vi "Ver 4.0.vi"() -> ()   [LabVIEW 2016]
doc: "This example VI shows how to use thermocouples to take a temperature measurement.\n\nNote:\nFor front panel measurements, make sure the Input switch is in the out position(F)\nFor plug-in card measurements, make sure the Input switch is in the in poisition(R)"
uses:
  Documents/keithley_27xx/Keithley 27XX/Public/Configure/Measurement Specific/Configure FRTD.vi
  Documents/keithley_27xx/Keithley 27XX/Public/Configure/Measurement Specific/Configure Thermocouple.vi
  Documents/keithley_27xx/Keithley 27XX/Public/Configure/Measurement Specific/Configure Thermistor.vi
  Documents/keithley_27xx/Keithley 27XX/Public/Data/Read Multiple Direct.vi
  Documents/keithley_27xx/Keithley 27XX/Keithley 27XX.lvlib
panel:
  out "XY Graph":cluster{dbl[], dbl[]}[](graph)
  out "Timestamp 2":dbl[](array[numeric])
  out "Timestamp 1":dbl[](array[numeric])
  out "Timestamp 0":dbl[](array[numeric])
  out "Case 2":dbl[](array[numeric])
  out "Case 1":dbl[](array[numeric])
  in  "Channel (2)":string="103"
  in  "Alpha2":dbl=0.0038
  in  "Beta2":dbl=0.1
  in  "Delta2 3":dbl=1.0
  in  "Sensor Type 2":string(combo)="Thermistor"
  in  "Channel (1)":string="102"
  in  "Alpha1":dbl=0.0038
  in  "Beta1":dbl=0.1
  in  "Delta1 2":dbl=1.0
  in  "Sensor Type 1":string(combo)="Thermistor"
  in  "Sensor Type 0":string(combo)="Thermistor"
  in  "Delta0":dbl=1.0
  in  "Beta0":dbl=0.1
  in  "Alpha0":dbl=0.0038
  in  "Serial Configuration":T1={"Baud Rate (9600)"=9600, "Flow Control (1: XON/XOFF)"=1, "Termination Char (0:CR)"=0} {"Termination Char (0:CR)" items=["CR", "LF", "CRLF (Do not use)", "LFCR (Do not use)"]; "Flow Control (1: XON/XOFF)" items=["None", "XON/XOFF", "RTS/CTS (2701 Only)", "XON/XOFF & RTS/CTS (2701 Only)"]; "Baud Rate (9600)" items=["300"=300, "600"=600, "1200"=1200, "2400"=2400, "4800"=4800, "9600"=9600, "19.2k"=19200, "38.4k (2701 Only)"=38400, "57.6k (2701 Only)"=57600, "115.2k (2701 Only)"=115200]}
  in  "VISA resource name":refnum<visa-resource-name>="TCPIP0::192.168.69.200::1394::SOCKET"
  in  "stop":bool
  out "Case 0":dbl[](array[numeric])
  in  "Channel (0)":string="101"
  in  "Temperature (0: Celsius)":u16(ring) items=["Celsius", "Fahrenheit", "Kelvin"]
  # "*For front panel measurements, make sure the Input switch is in the out position(F)*\n  For plug-in card measurements, make sure the Input switch is in the in position(R)"
  # "© 2005 National Instruments Corporation.  ALL RIGHTS RESERVED."
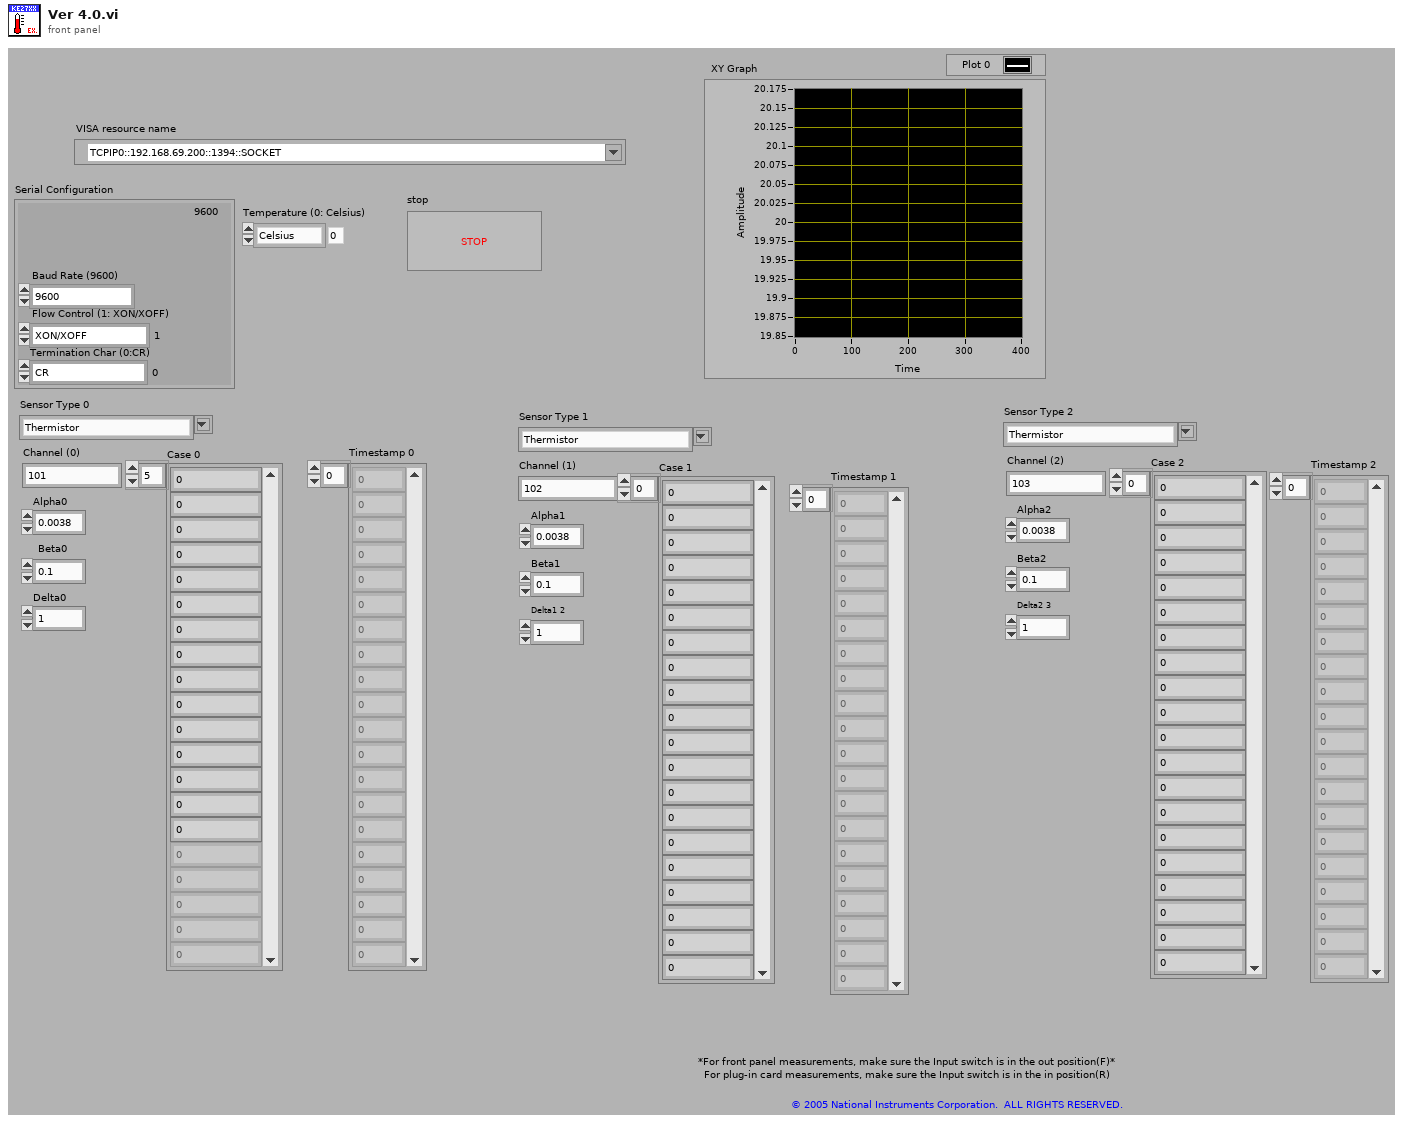
[diagram p1: front panel]
types:
  T1 = cluster{"Baud Rate (9600)":u32, "Flow Control (1: XON/XOFF)":u16, "Termination Char (0:CR)":u16}
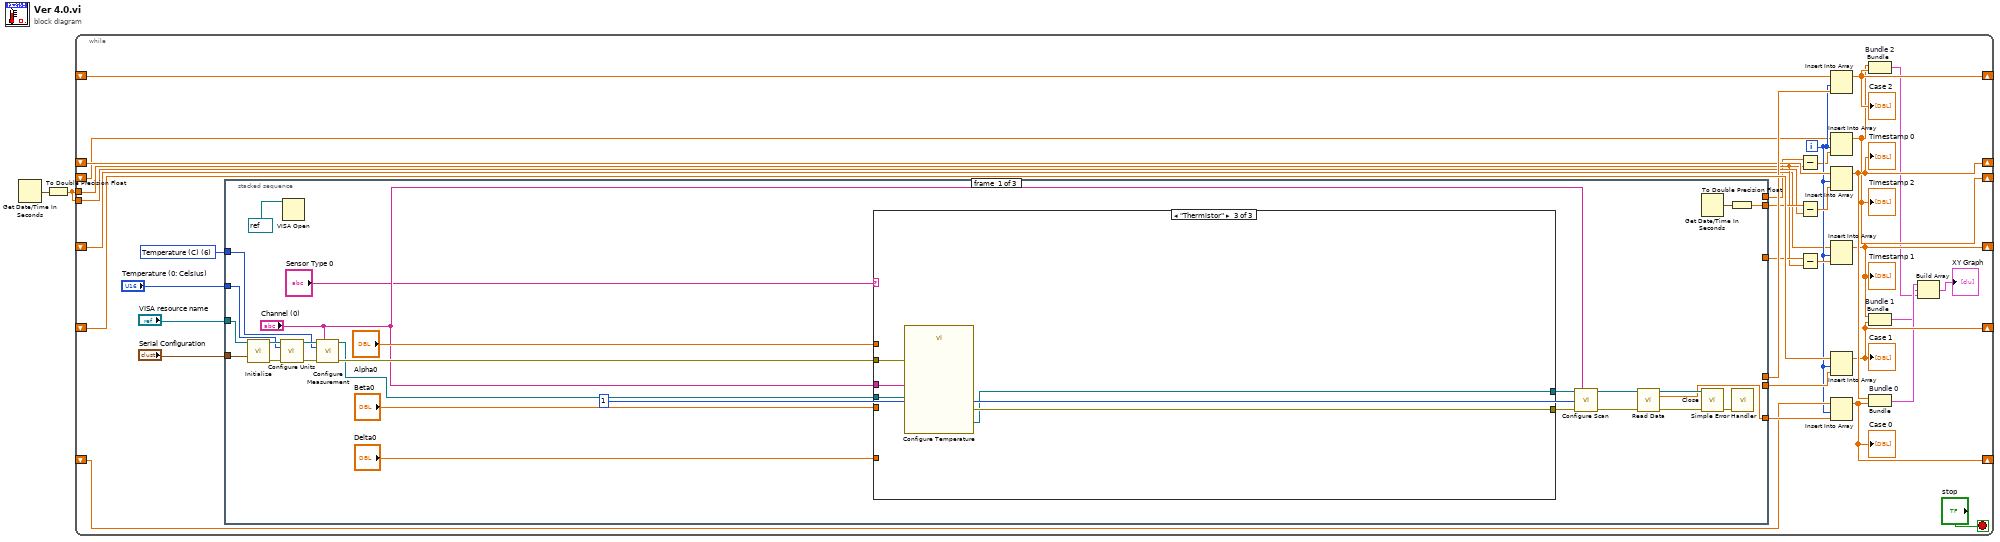
[diagram p0: block diagram]
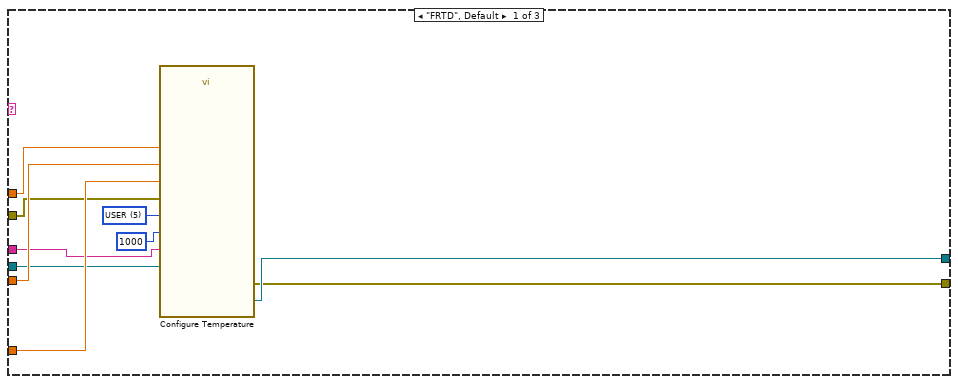
[diagram p2: hidden frame]
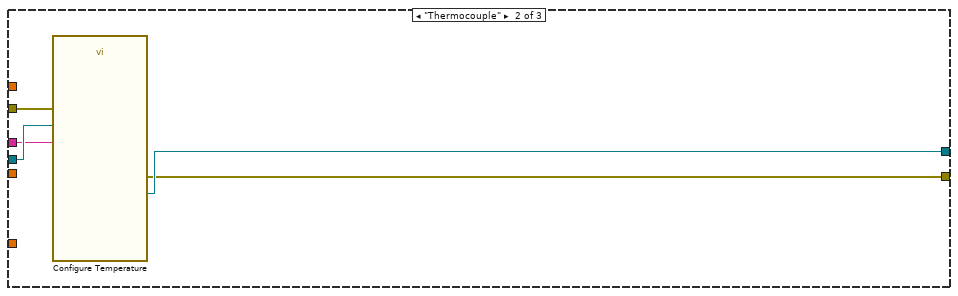
[diagram p3: hidden frame]
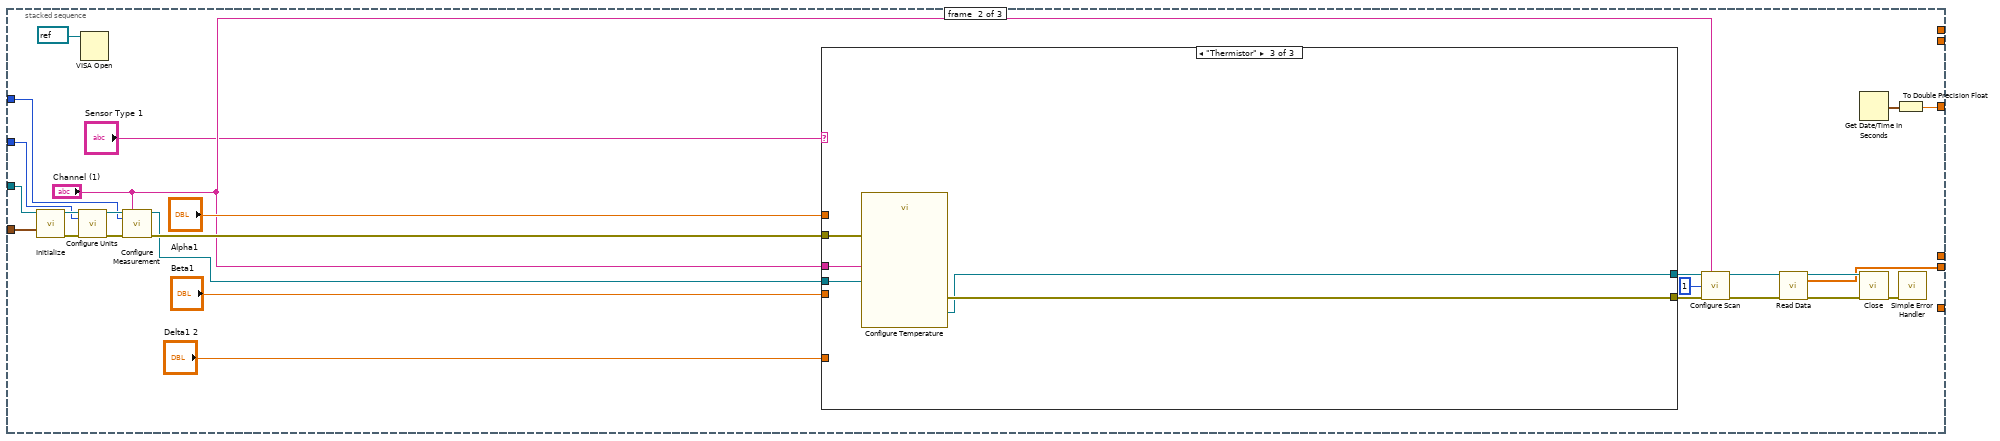
[diagram p4: hidden frame]
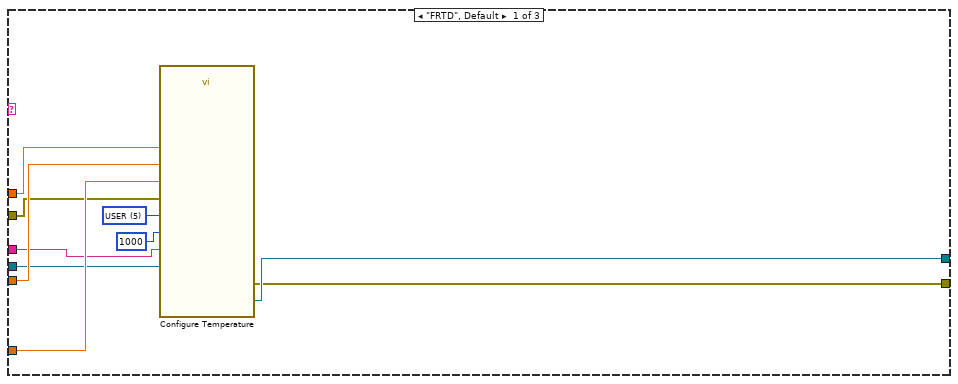
[diagram p5: hidden frame]
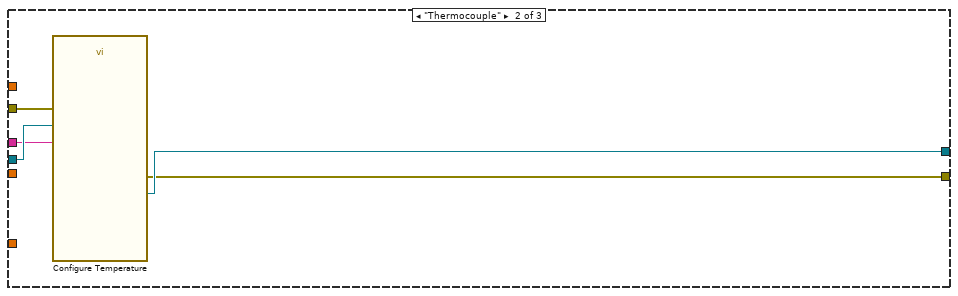
[diagram p6: hidden frame]
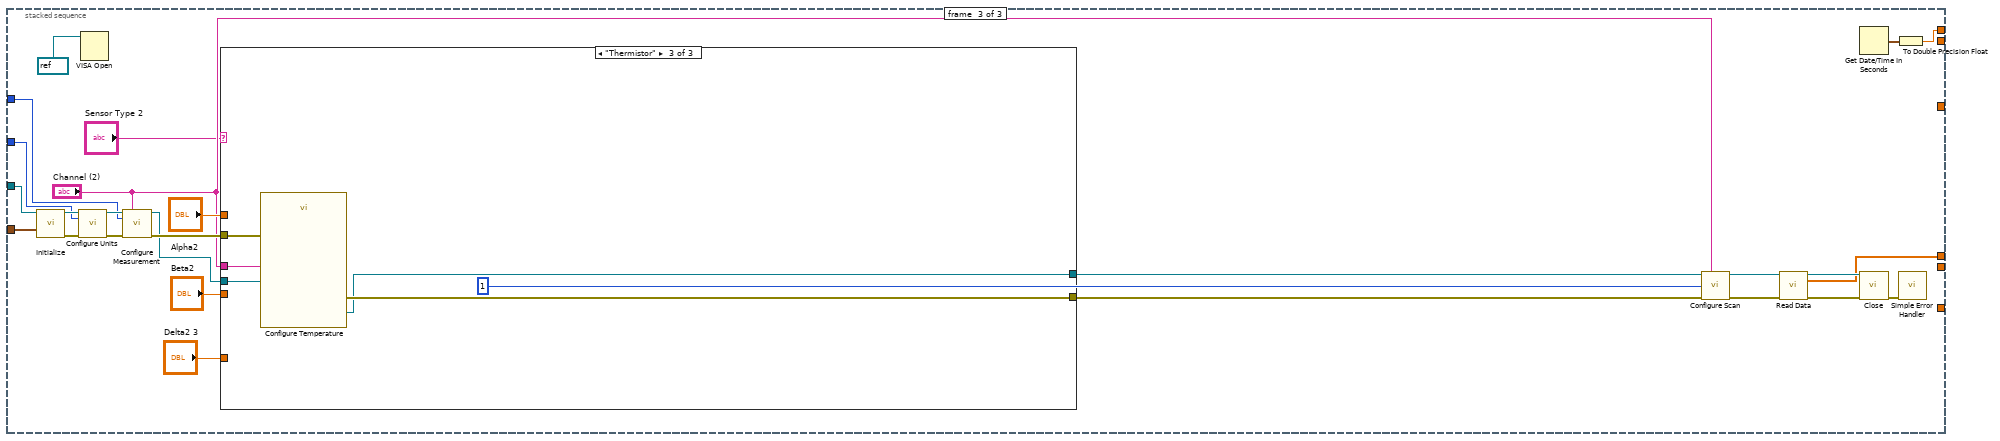
[diagram p7: hidden frame]
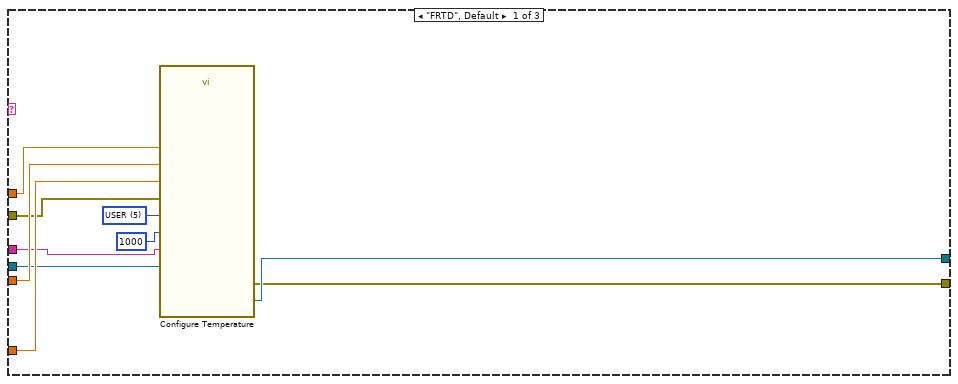
[diagram p8: hidden frame]
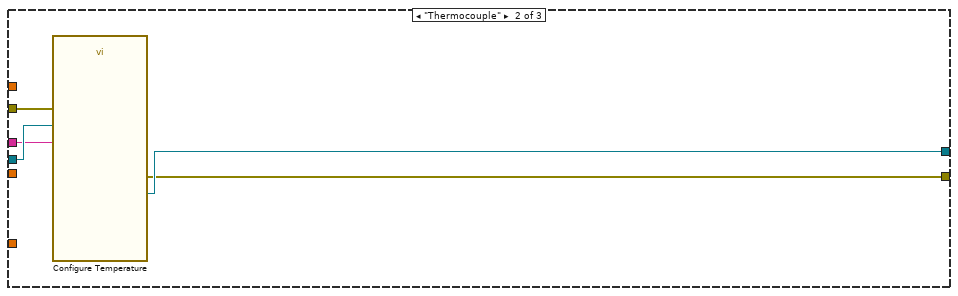
[diagram p9: hidden frame]
diagram:
  n1 = Get Date/Time In Seconds() -> (seconds since 1Jan1904=w2:timestamp)
  n2 = To Double Precision Float(number=w2) -> (double precision float=w1:dbl)
  n3 = while {
    shift-right: [w20] -> _
    shift-left: _ -> [w29]
    shift-right: [w11] -> _
    shift-left: _ -> [w27]
    shift-right: [w10] -> _
    shift-left: _ -> [w25]
    tunnel: w1 -> [w23]
    shift-right: [w19] -> _
    shift-left: _ -> [w21]
    tunnel: w1 -> [w17]
    shift-right: [w12] -> _
    shift-left: _ -> [w13]
    shift-right: [w9] -> _
    shift-left: _ -> [w8]
    i -> [w15]
    stop <- "stop" stop-if-true
    w33 = u16 6 items=["DC Voltage", "AC Voltage", "DC Current", "AC Current", "Resistance", "Four-Wire Resistance", "Temperature (C)", "Frequency", "Period", "Continuity"] ("Function (0: DC Voltage)")
    n4 = stacked-sequence {
      tunnel: "VISA resource name" -> [w52 w99 w146]
      tunnel: "Serial Configuration" -> [w51 w98 w145]
      tunnel: w33 -> [w50 w97 w144]
      tunnel: "Temperature (0: Celsius)" -> [w49 w96 w143]
      tunnel: [w38 _ _] -> w31
      tunnel: [_ w85 _] -> w28
      tunnel: [_ _ w132] -> w26
      tunnel: [w36 _ _] -> w24
      tunnel: [_ w83 _] -> w18
      tunnel: [_ _ w130] -> w7
      frame #0 {
        n5 = call "Initialize.vi"("VISA resource name"=w52, "Serial Configuration"=w51) -> ("VISA resource name out"=w61:refnum<visa-resource-name>, "error out"=w55:errorcluster)  [unwired: 12 in]
        n6 = call "Configure Units.vi"("VISA resource name"=w61, "Temperature (0: Celsius)"=w49, "error in (no error)"=w55) -> ("VISA resource name out"=w62:refnum<visa-resource-name>, "error out"=w54:errorcluster)  [unwired: 11 in]
        n7 = VISA Open(VISA resource name=refnum<visa-resource-name> refnum) -> ()  [unwired: 4 in, 2 out]
        n8 = call "Configure Measurement.vi"("VISA resource name"=w62, "Scan List (Empty)"="Channel (0)", "Function (0: DC Voltage)"=w50, "error in (no error)"=w54) -> ("VISA resource name out"=w42:refnum<visa-resource-name>, "error out"=w43:errorcluster)  [unwired: 10 in]
        n9 = case shown="\"Thermistor\"" "Sensor Type 0" {
          tunnel: [w71 w76 w82] -> w48
          tunnel: [w72 w77 w81] -> w47
          tunnel: "Delta0" -> [w66 _ _]
          tunnel: "Beta0" -> [w67 _ _]
          tunnel: "Alpha0" -> [w68 _ _]
          tunnel: w43 -> [w65 w75 w78]
          tunnel: w42 -> [w64 w74 w79]
          tunnel: "Channel (0)" -> [w63 w73 w80]
          frame "FRTD", Default {
            w70 = u16 5 items=["PT100", "D100", "F100", "PT3916", "PT385", "USER"] ("FRTD Type (0: PT100)")
            n10 = call-poly "Configure Temperature.vi"("VISA resource name"=w64, "FRTD Type (0: PT100)"=w70, "error in (no error)"=w65, "Scan List (Empty)"=w63, "R Zero (100)"=1000, "Alpha (0.00385)"=w68, "Beta (0.111)"=w67, "Delta (1.507)"=w66) -> ("VISA resource name out"=w72:refnum<visa-resource-name>, "error out"=w71:errorcluster)  [unwired: 10 in]
          }
          frame "Thermocouple" {
            n11 = call-poly "Configure Temperature.vi"("VISA resource name"=w74, "error in (no error)"=w75, "Scan List (Empty)"=w73) -> ("VISA resource name out"=w77:refnum<visa-resource-name>, "error out"=w76:errorcluster)  [unwired: 15 in]
          }
          frame "Thermistor" {
            n12 = call-poly "Configure Temperature.vi"("VISA resource name"=w79, "error in (no error)"=w78, "Scan List (Empty)"=w80) -> ("VISA resource name out"=w81:refnum<visa-resource-name>, "error out"=w82:errorcluster)  [unwired: 15 in]
          }
        }
        n13 = call "Configure Scan.vi"("VISA resource name"=w47, "Channel List (101:110)"="Channel (0)", "Sample Count (100)"=1, "error in (no error)"=w48) -> ("VISA resource name out"=w58:refnum<visa-resource-name>, "error out"=w59:errorcluster)  [unwired: 10 in]
        n14 = call-poly "Read Data.vi"("VISA resource name"=w58, "error in (no error)"=w59) -> ("VISA resource name out"=w56:refnum<visa-resource-name>, "Measurement Data"=w38:dbl[], "error out"=w57:errorcluster)  [unwired: 8 in, 3 out]
        n15 = Get Date/Time In Seconds() -> (seconds since 1Jan1904=w37:timestamp)
        n16 = call "Close.vi"("VISA resource name"=w56, "error in (no error)"=w57) -> ("error out"=w60:errorcluster)  [unwired: 13 in]
        n17 = To Double Precision Float(number=w37) -> (double precision float=w36:dbl)
        n18 = call <vilib>:"Simple Error Handler.vi"("error in (no error)"=w60) -> ()  [unwired: 4 in, 5 out]
      }
      frame #1 {
        n19 = call "Initialize.vi"("VISA resource name"=w99, "Serial Configuration"=w98) -> ("VISA resource name out"=w108:refnum<visa-resource-name>, "error out"=w102:errorcluster)  [unwired: 12 in]
        n20 = call "Configure Units.vi"("VISA resource name"=w108, "Temperature (0: Celsius)"=w96, "error in (no error)"=w102) -> ("VISA resource name out"=w109:refnum<visa-resource-name>, "error out"=w101:errorcluster)  [unwired: 11 in]
        n21 = VISA Open(VISA resource name=refnum<visa-resource-name> refnum) -> ()  [unwired: 4 in, 2 out]
        n22 = call "Configure Measurement.vi"("VISA resource name"=w109, "Scan List (Empty)"="Channel (1)", "Function (0: DC Voltage)"=w97, "error in (no error)"=w101) -> ("VISA resource name out"=w89:refnum<visa-resource-name>, "error out"=w90:errorcluster)  [unwired: 10 in]
        n23 = case shown="\"Thermistor\"" "Sensor Type 1" {
          tunnel: [w118 w123 w129] -> w95
          tunnel: [w119 w124 w128] -> w94
          tunnel: "Delta1 2" -> [w113 _ _]
          tunnel: "Beta1" -> [w114 _ _]
          tunnel: "Alpha1" -> [w115 _ _]
          tunnel: w90 -> [w112 w122 w125]
          tunnel: w89 -> [w111 w121 w126]
          tunnel: "Channel (1)" -> [w110 w120 w127]
          frame "FRTD", Default {
            w117 = u16 5 items=["PT100", "D100", "F100", "PT3916", "PT385", "USER"] ("FRTD Type (0: PT100)")
            n24 = call-poly "Configure Temperature.vi"("VISA resource name"=w111, "FRTD Type (0: PT100)"=w117, "error in (no error)"=w112, "Scan List (Empty)"=w110, "R Zero (100)"=1000, "Alpha (0.00385)"=w115, "Beta (0.111)"=w114, "Delta (1.507)"=w113) -> ("VISA resource name out"=w119:refnum<visa-resource-name>, "error out"=w118:errorcluster)  [unwired: 10 in]
          }
          frame "Thermocouple" {
            n25 = call-poly "Configure Temperature.vi"("VISA resource name"=w121, "error in (no error)"=w122, "Scan List (Empty)"=w120) -> ("VISA resource name out"=w124:refnum<visa-resource-name>, "error out"=w123:errorcluster)  [unwired: 15 in]
          }
          frame "Thermistor" {
            n26 = call-poly "Configure Temperature.vi"("VISA resource name"=w126, "error in (no error)"=w125, "Scan List (Empty)"=w127) -> ("VISA resource name out"=w128:refnum<visa-resource-name>, "error out"=w129:errorcluster)  [unwired: 15 in]
          }
        }
        n27 = call "Configure Scan.vi"("VISA resource name"=w94, "Channel List (101:110)"="Channel (1)", "Sample Count (100)"=1, "error in (no error)"=w95) -> ("VISA resource name out"=w105:refnum<visa-resource-name>, "error out"=w106:errorcluster)  [unwired: 10 in]
        n28 = call-poly "Read Data.vi"("VISA resource name"=w105, "error in (no error)"=w106) -> ("VISA resource name out"=w103:refnum<visa-resource-name>, "Measurement Data"=w85:dbl[], "error out"=w104:errorcluster)  [unwired: 8 in, 3 out]
        n29 = Get Date/Time In Seconds() -> (seconds since 1Jan1904=w84:timestamp)
        n30 = call "Close.vi"("VISA resource name"=w103, "error in (no error)"=w104) -> ("error out"=w107:errorcluster)  [unwired: 13 in]
        n31 = To Double Precision Float(number=w84) -> (double precision float=w83:dbl)
        n32 = call <vilib>:"Simple Error Handler.vi"("error in (no error)"=w107) -> ()  [unwired: 4 in, 5 out]
      }
      frame #2 {
        n33 = call "Initialize.vi"("VISA resource name"=w146, "Serial Configuration"=w145) -> ("VISA resource name out"=w155:refnum<visa-resource-name>, "error out"=w149:errorcluster)  [unwired: 12 in]
        n34 = call "Configure Units.vi"("VISA resource name"=w155, "Temperature (0: Celsius)"=w143, "error in (no error)"=w149) -> ("VISA resource name out"=w156:refnum<visa-resource-name>, "error out"=w148:errorcluster)  [unwired: 11 in]
        n35 = VISA Open(VISA resource name=refnum<visa-resource-name> refnum) -> ()  [unwired: 4 in, 2 out]
        n36 = call "Configure Measurement.vi"("VISA resource name"=w156, "Scan List (Empty)"="Channel (2)", "Function (0: DC Voltage)"=w144, "error in (no error)"=w148) -> ("VISA resource name out"=w136:refnum<visa-resource-name>, "error out"=w137:errorcluster)  [unwired: 10 in]
        n37 = case shown="\"Thermistor\"" "Sensor Type 2" {
          tunnel: [w165 w170 w176] -> w142
          tunnel: [w166 w171 w175] -> w141
          tunnel: "Delta2 3" -> [w160 _ _]
          tunnel: "Beta2" -> [w161 _ _]
          tunnel: "Alpha2" -> [w162 _ _]
          tunnel: w137 -> [w159 w169 w172]
          tunnel: w136 -> [w158 w168 w173]
          tunnel: "Channel (2)" -> [w157 w167 w174]
          frame "FRTD", Default {
            w164 = u16 5 items=["PT100", "D100", "F100", "PT3916", "PT385", "USER"] ("FRTD Type (0: PT100)")
            n38 = call-poly "Configure Temperature.vi"("VISA resource name"=w158, "FRTD Type (0: PT100)"=w164, "error in (no error)"=w159, "Scan List (Empty)"=w157, "R Zero (100)"=1000, "Alpha (0.00385)"=w162, "Beta (0.111)"=w161, "Delta (1.507)"=w160) -> ("VISA resource name out"=w166:refnum<visa-resource-name>, "error out"=w165:errorcluster)  [unwired: 10 in]
          }
          frame "Thermocouple" {
            n39 = call-poly "Configure Temperature.vi"("VISA resource name"=w168, "error in (no error)"=w169, "Scan List (Empty)"=w167) -> ("VISA resource name out"=w171:refnum<visa-resource-name>, "error out"=w170:errorcluster)  [unwired: 15 in]
          }
          frame "Thermistor" {
            n40 = call-poly "Configure Temperature.vi"("VISA resource name"=w173, "error in (no error)"=w172, "Scan List (Empty)"=w174) -> ("VISA resource name out"=w175:refnum<visa-resource-name>, "error out"=w176:errorcluster)  [unwired: 15 in]
          }
        }
        n41 = call "Configure Scan.vi"("VISA resource name"=w141, "Channel List (101:110)"="Channel (2)", "Sample Count (100)"=1, "error in (no error)"=w142) -> ("VISA resource name out"=w152:refnum<visa-resource-name>, "error out"=w153:errorcluster)  [unwired: 10 in]
        n42 = call-poly "Read Data.vi"("VISA resource name"=w152, "error in (no error)"=w153) -> ("VISA resource name out"=w150:refnum<visa-resource-name>, "Measurement Data"=w132:dbl[], "error out"=w151:errorcluster)  [unwired: 8 in, 3 out]
        n43 = Get Date/Time In Seconds() -> (seconds since 1Jan1904=w131:timestamp)
        n44 = call "Close.vi"("VISA resource name"=w150, "error in (no error)"=w151) -> ("error out"=w154:errorcluster)  [unwired: 13 in]
        n45 = To Double Precision Float(number=w131) -> (double precision float=w130:dbl)
        n46 = call <vilib>:"Simple Error Handler.vi"("error in (no error)"=w154) -> ()  [unwired: 4 in, 5 out]
      }
    }
    n47 = Subtract(x=w7, y=w17) -> (x-y=w14:dbl)
    n48 = Subtract(x=w24, y=w23) -> (x-y=w22:dbl)
    n49 = Subtract(x=w18, y=w17) -> (x-y=w16:dbl)
    n50 = Insert Into Array(array=w25, index=w15, new element=w26) -> (w10:dbl[])
    "Case 2" <- w10
    n51 = Insert Into Array(array=w8, index=w15, new element=w14) -> (w9:dbl[])
    "Timestamp 2" <- w9
    n52 = Insert Into Array(array=w21, index=w15, new element=w22) -> (w19:dbl[])
    "Timestamp 0" <- w19
    n53 = Insert Into Array(array=w13, index=w15, new element=w16) -> (w12:dbl[])
    "Timestamp 1" <- w12
    n54 = Insert Into Array(array=w27, index=w15, new element=w28) -> (w11:dbl[])
    "Case 1" <- w11
    n55 = Insert Into Array(array=w29, index=w15, new element=w31) -> (w20:dbl[])
    "Case 0" <- w20
    n56 = Bundle "Bundle 2"(w9, w10) -> (w4:cluster{dbl[], dbl[]})  [unwired: 1 in]
    n57 = Bundle "Bundle 1"(w12, w11) -> (w5:cluster{dbl[], dbl[]})  [unwired: 1 in]
    n58 = Bundle "Bundle 0"(w19, w20) -> (w6:cluster{dbl[], dbl[]})  [unwired: 1 in]
    n59 = Build Array(w6, w5, w4) -> (→"XY Graph":cluster{dbl[], dbl[]}[])
  }
